vi "F60_Diagnostic.vi"() -> (2 "Edit BSA Setup Out":bool)   [LabVIEW 2010]
uses:
  Globals/LDA_meas_global_1.vi
  Globals/LDA_meas_global_2.vi
panel:
  out "Data 2":dbl[](graph)
  in  "Configuration":string(combo)="0"
  in  "samples":i32=500
  in  "time (s)":sgl=5.0
  in  "Edit BSA Setup":bool
  out "Data":dbl[](graph)
  in  "Start ACQ":bool
  in  "stop":bool
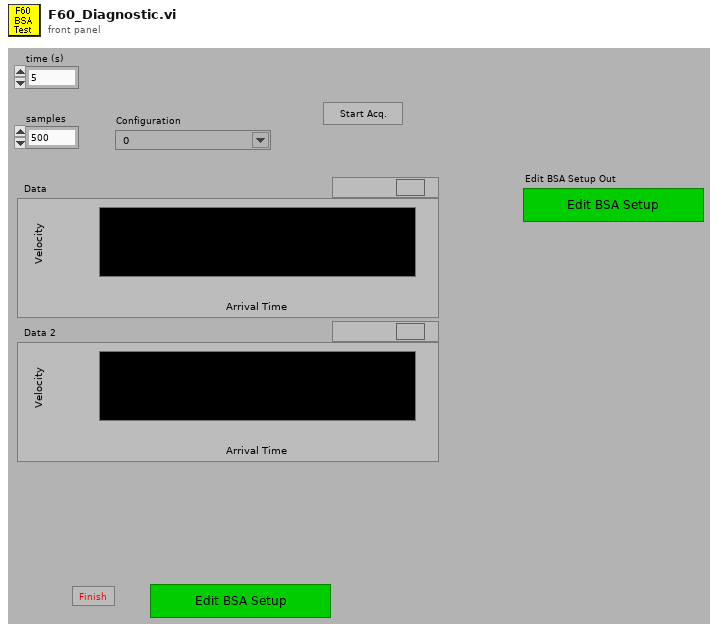
[diagram p1: front panel]
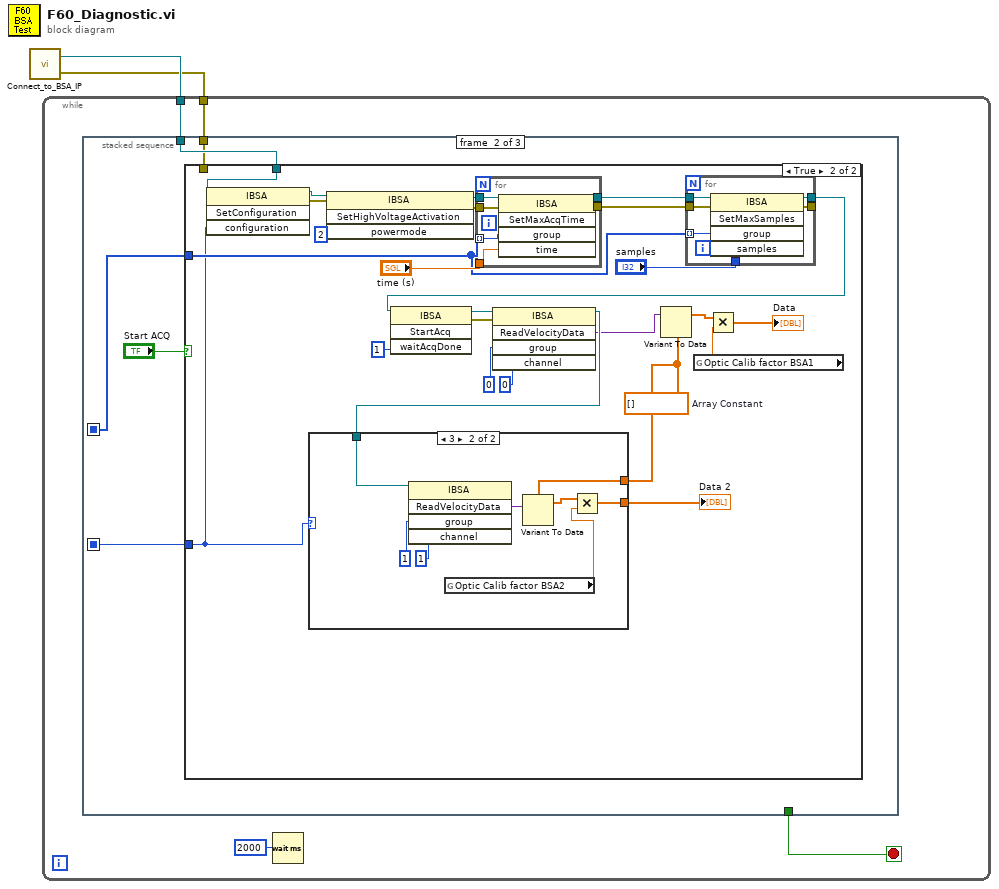
[diagram p0: block diagram]
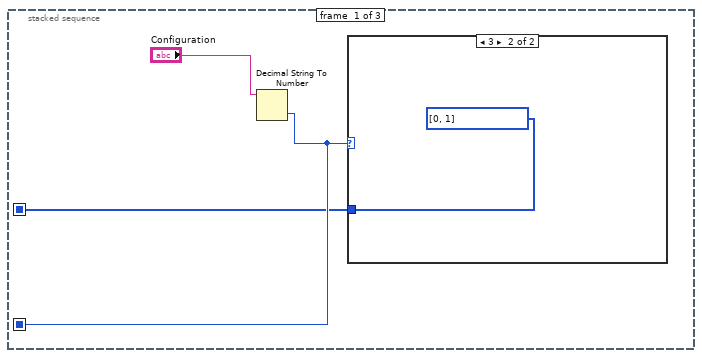
[diagram p2: hidden frame]
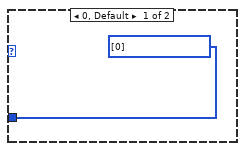
[diagram p3: hidden frame]
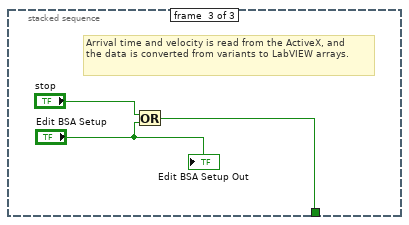
[diagram p6: hidden frame]
diagram:
  n1 = call "Connect_to_BSA_IP.vi"() -> ("error out"=w1:errorcluster, "BSA"=w2:refnum<k7>)  [unwired: 2 out]
  n2 = while {
    tunnel: w2 -> [w6]
    tunnel: w1 -> [w5]
    stop <- w4 stop-if-true
    n3 = stacked-sequence {
      seq-local: [w8 _ _] -> [_ w12 _]
      seq-local: [w7 _ _] -> [_ w13 _]
      tunnel: w6 -> [_ w15 _]
      tunnel: w5 -> [_ w14 _]
      tunnel: [_ _ w65] -> w4
      frame #0 {
        n4 = Decimal String To Number(string="Configuration") -> (number=w8:i32)  [unwired: 3 out]
        n5 = case shown="3" w8 {
          tunnel: [i32[] [0] i32[] [0, 1]] -> w7
          frame 0, Default {
          }
          frame 3 {
          }
        }
      }
      frame #1 {
        n6 = case shown="True" "Start ACQ" {
          tunnel: w15 -> [_ w21]
          tunnel: w14 -> [_ _]
          tunnel: w13 -> [_ w23]
          tunnel: w12 -> [_ w20]
          frame False {
          }
          frame True {
            w26 = dbl[] []  # Array Constant
            n7 = invoke class="IBSA" method="SetConfiguration"(reference=w21, "configuration"=w20) -> (reference out=w18:refnum<k7>, error out=w17:errorcluster)  [unwired: 2 in, 2 out]
            n8 = invoke class="IBSA" method="SetHighVoltageActivation"(reference=w18, error in=w17, "powermode"=2) -> (reference out=w40:refnum<k7>, error out=w41:errorcluster)  [unwired: 1 in, 2 out]
            n9 = for {
              tunnel: w41 -> [w53]
              tunnel: w40 -> [w52]
              tunnel: "time (s)" -> [w51]
              tunnel: [w50] -> w38
              tunnel: [w49] -> w37
              tunnel: w23 -> [w48] mode=indexing
              n10 = invoke class="IBSA" method="SetMaxAcqTime"(reference=w52, error in=w53, "group"=w48, "time"=w51) -> (reference out=w50:refnum<k7>, error out=w49:errorcluster)  [unwired: 1 in, 3 out]
            }
            n11 = for {
              tunnel: w23 -> [w47] mode=indexing
              tunnel: w38 -> [w46]
              tunnel: w37 -> [w45]
              tunnel: "samples" -> [w44]
              tunnel: [w43] -> w19
              tunnel: [w42] -> _
              n12 = invoke class="IBSA" method="SetMaxSamples"(reference=w46, error in=w45, "group"=w47, "samples"=w44) -> (reference out=w43:refnum<k7>, error out=w42:errorcluster)  [unwired: 1 in, 3 out]
            }
            n13 = invoke class="IBSA" method="StartAcq"(reference=w19, "waitAcqDone"=1) -> (reference out=w31:refnum<k7>, error out=w32:errorcluster)  [unwired: 2 in, 2 out]
            n14 = invoke class="IBSA" method="ReadVelocityData"(reference=w31, error in=w32, "group"=0, "channel"=0 ("ich")) -> (reference out=w27:refnum<k7>, "ReadVelocityData"=w24:variant)  [unwired: 1 in, 3 out]
            n15 = case shown="3" w20 {
              tunnel: w27 -> [_ w60]
              tunnel: w26 -> [w54 w59]
              tunnel: [w54 w56] -> w25
              frame 0, Default {
              }
              frame 3 {
                n16 = invoke class="IBSA" method="ReadVelocityData"(reference=w60, "group"=1, "channel"=1 ("ich")) -> ("ReadVelocityData"=w58:variant)  [unwired: 2 in, 4 out]
                n17 = global read "LDA_meas_global_2.vi" "Optic Calib factor BSA2"() -> (w55:dbl)
                n18 = Variant To Data(Variant=w58, type=w59) -> (data=w57:dbl[])  [unwired: 1 in, 1 out]
                n19 = Multiply(x=w57, y=w55) -> (x*y=w56:dbl[])
              }
            }
            "Data 2" <- w25
            n20 = Variant To Data(Variant=w24, type=w26) -> (data=w29:dbl[])  [unwired: 1 in, 1 out]
            n21 = global read "LDA_meas_global_1.vi" "Optic Calib factor BSA1"() -> (w30:dbl)
            n22 = Multiply(x=w29, y=w30) -> (x*y=→"Data":dbl[])
          }
        }
      }
      frame #2 {
        # "Arrival time and velocity is read from the ActiveX, and \nthe data is converted from variants to LabVIEW arrays."
        n23 = Or(x="stop", y="Edit BSA Setup") -> (x .or. y?=w65:bool)
        "Edit BSA Setup Out" <- "Edit BSA Setup"
      }
    }
    n24 = Wait (ms)(milliseconds to wait=u32 2000) -> ()  [unwired: 1 out]
  }
